vi "setSpeed.vi"(8 "error in":errorcluster, 11 "Speed":bool) -> (0 "error out":errorcluster)   [LabVIEW 2024]
doc: "Funkcja służąca do sterowania wentylatorem w symulowanym piekarniku. Wartość TRUE wejścia włącza wentylator, wartość FALSE wejścia wyłącza wentylator."
uses:
  TypeDefs/Heater_interface.ctl
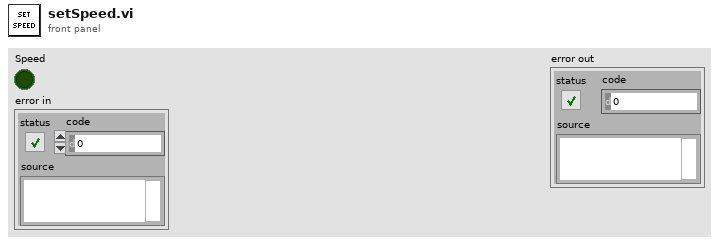
[diagram p1: front panel]
types:
  T1 = typedef "Heater_interface.ctl" = enum16{"setSpeed", "setHeaters", "getTemperature"}
  T2 = cluster{"Interface":T1, "Parameter1":variant, "Parameter2":variant}
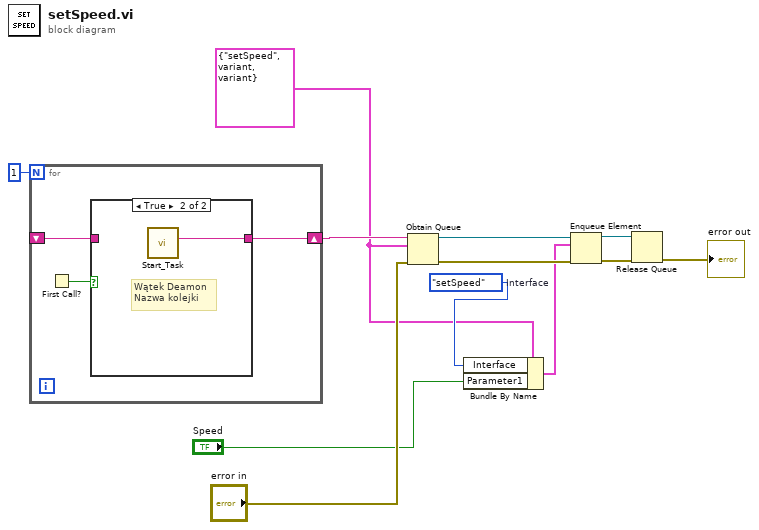
[diagram p0: block diagram]
diagram:
  w2 = T2 {"Interface"=enum."setSpeed", "Parameter1"=variant, "Parameter2"=variant}
  w3 = Heater_interface."setSpeed"  # Interface
  n1 = for {
    N: 1 -> [_]
    shift-right: [w14] -> w11
    shift-left: _ -> [w13]
    n2 = First Call?() -> (First Call?: T/F=w15:bool)
    n3 = case shown="True" w15 {
      tunnel: [w16 w17] -> w14
      tunnel: w13 -> [w16 _]
      frame False {
      }
      frame True {
        # "Wątek Deamon\nNazwa kolejki"
        n4 = call "Start_Task.vi"() -> ("QueueName"=w17:string)  [unwired: 11 in]
      }
    }
  }
  n5 = Obtain Queue(name (unnamed)=w11, element data type=w2, error in (no error)="error in") -> (queue out=w10:refnum<queue>, error out=w9:errorcluster)  [unwired: 2 in, 1 out]
  n6 = Bundle By Name(cluster=w2, "Interface"=w3, "Parameter1"="Speed") -> (w8:T2)
  n7 = Enqueue Element(queue=w10, element=w8, error in (no error)=w9) -> (queue out=w7:refnum<queue>, error out=w6:errorcluster)  [unwired: 1 in, 1 out]
  n8 = Release Queue(queue=w7, error in (no error)=w6) -> (error out=→"error out":errorcluster)  [unwired: 1 in, 2 out]
